vi "SetParam.vi"(8 "error in (no error)":errorcluster caption="entrée d'erreur (pas d'erreur)", 10 "mutual_info_score":T1, 11 "Mutual_Info_Score.lvclass":refnum<class "Mutual_Info_Score.lvclass">) -> (0 "error out":errorcluster caption="sortie d'erreur", 3 "Mutual_Info_Score.lvclass":refnum<class "Mutual_Info_Score.lvclass">)   [LabVIEW 2020, in "Mutual_Info_Score.lvclass"]
doc: "Set Parameters"
uses:
  Mutual_Info_Score.lvclass
  Mutual_Info_Score.lvclass/Mutual_Info_Score.ctl
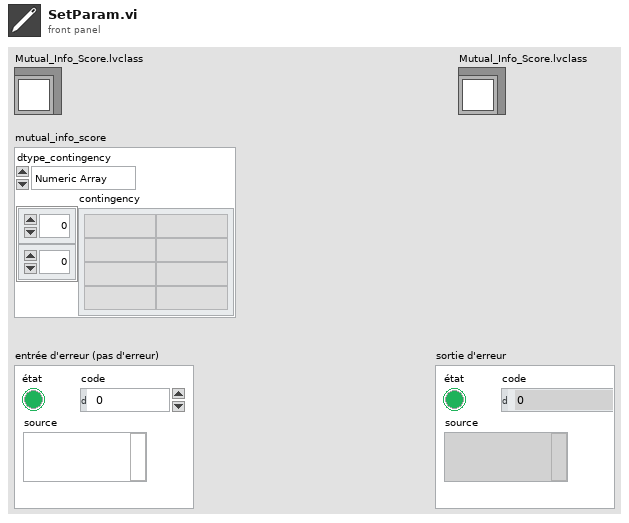
[diagram p1: front panel]
types:
  T1 = cluster{"dtype_contingency":enum16{"Numeric Array", "String Array", "Sparse"}, "contingency":string[][]}
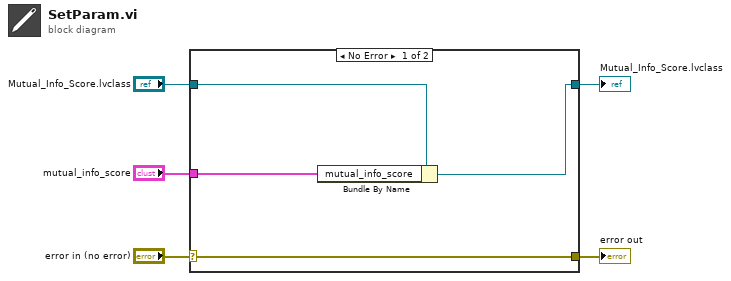
[diagram p0: block diagram]
diagram:
  n1 = case shown="No Error" "error in (no error)" {
    selector: "error in (no error)" -> [w9 w10]
    tunnel: [w9 w10] -> w4
    tunnel: [w7 w11] -> w2
    tunnel: "Mutual_Info_Score.lvclass" -> [w8 w11]
    tunnel: "mutual_info_score" -> [w6 _]
    frame No Error {
      n2 = Bundle By Name(cluster=w8, "mutual_info_score"=w6) -> (w7:refnum<class "Mutual_Info_Score.lvclass">)
    }
    frame Error {
    }
  }
  "error out" <- w4
  "Mutual_Info_Score.lvclass" <- w2
